vi "Set__slk_mt.vi"(7 "values":string[][](array[string]), 8 "error in (no error)":errorcluster, 11 "digital u32 in":refnum<class "Digital U32__slk_mt.lvclass">) -> (0 "error out":errorcluster, 3 "digital u32 out":refnum<class "Digital U32__slk_mt.lvclass">)   [LabVIEW 2014, in "Lazyboots Menu Tool.lvlib" / "Digital U32__slk_mt.lvclass"]
doc: "Sets the values to the control on GUI.\n\n<b>Values:</b>\n[ [Section, Key, Value], [Section, Key, Value], ..., [Section, Key, Value] ]"
uses:
  Digital U32__slk_mt.lvclass
  Digital U32__slk_mt.lvclass/Digital U32__slk_mt.ctl
panel:
  # "Set__slk_mt.vi\nSets the values to the control on GUI.\n\nNOTICE -- YOU MUST LEAVE THIS NOTICE IN PLACE.\n\nCopyright (c) 2011, LIANG LIU Shawn.Liu.cn@gmail.com\nAll rights reserved.\n\nRedistribution and use in source and binary forms, with or without modification, are permitted provided that the following conditions are met:\n-Redistributions of source code must retain the above copyright notice, this list of conditions and the following disclaimer.\n-Redistributions in binary form must reproduce the above copyright notice, this list of conditions and the following disclaimer in the documentation and/or other materials provided with the distribution.\n-Neither the name of the eLp nor the names of its contributors may be used to endorse or promote products derived from this software without specific prior written permission.\n\nTHIS SOFTWARE IS PROVIDED BY THE COPYRIGHT HOLDERS AND CONTRIBUTORS \"AS IS\" AND ANY EXPRESS OR IMPLIED WARRANTIES, INCLUDING, BUT NOT LIMITED TO, THE IMPLIED WARRANTIES OF MERCHANTABILITY AND FITNESS FOR A PARTICULAR PURPOSE ARE DISCLAIMED. IN NO EVENT SHALL THE COPYRIGHT HOLDER OR CONTRIBUTORS BE LIABLE FOR ANY DIRECT, INDIRECT, INCIDENTAL, SPECIAL, EXEMPLARY, OR CONSEQUENTIAL DAMAGES (INCLUDING, BUT NOT LIMITED TO, PROCUREMENT OF SUBSTITUTE GOODS OR SERVICES; LOSS OF USE, DATA, OR PROFITS; OR BUSINESS INTERRUPTION) HOWEVER CAUSED AND ON ANY THEORY OF LIABILITY, WHETHER IN CONTRACT, STRICT LIABILITY, OR TORT (INCLUDING NEGLIGENCE OR OTHERWISE) ARISING IN ANY WAY OUT OF THE USE OF THIS SOFTWARE, EVEN IF ADVISED OF THE POSSIBILITY OF SUCH DAMAGE."
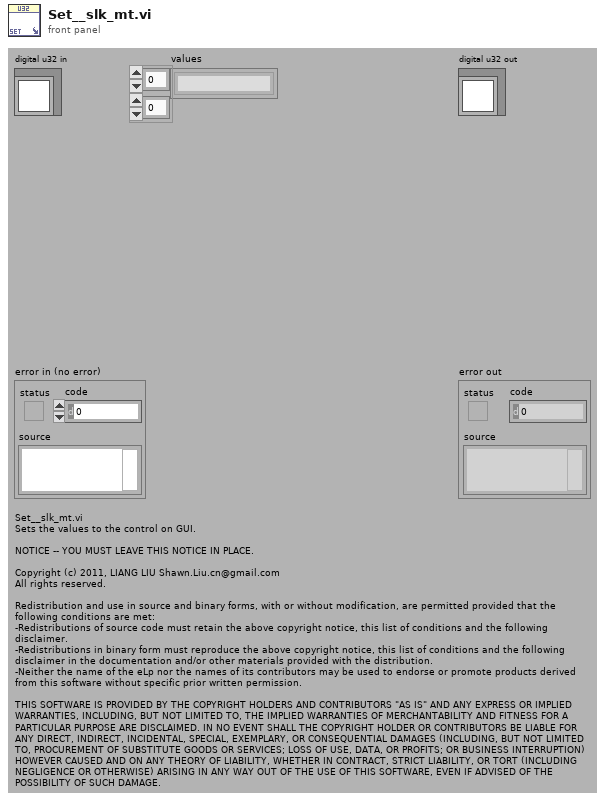
[diagram p1: front panel]
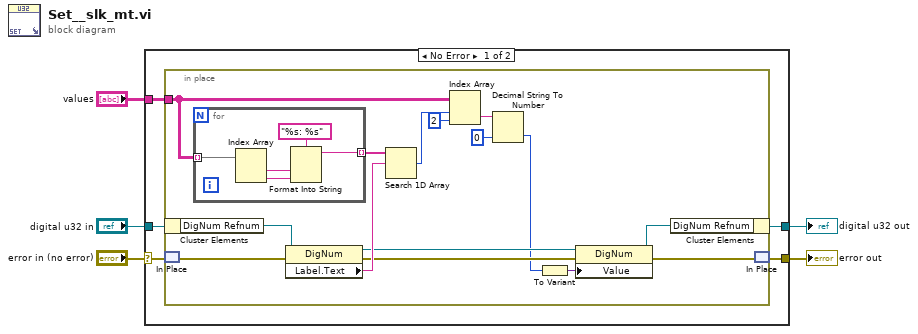
[diagram p0: block diagram]
diagram:
  n1 = case shown="No Error" "error in (no error)" {
    selector: "error in (no error)" -> [w8 w32]
    tunnel: "values" -> [w10 _]
    tunnel: "digital u32 in" -> [w9 w31]
    tunnel: [w7 w32] -> w2
    tunnel: [w6 w31] -> w1
    frame No Error {
      n2 = in-place {
        in-place-border: w10 -> [w15]
        n3 = in-place-cluster #1(w9) -> ("DigNum Refnum"=w14:refnum<vi>)
        n4 = in-place-match #2(w8) -> (w11:errorcluster)
        n5 = for {
          tunnel: w15 -> [w30] mode=indexing
          tunnel: [w26] -> w25 mode=indexing
          n6 = Index Array(array=w30) -> (element #1=w28:string, element #2=w27:string)  [unwired: 2 in]
          n7 = Format Into String(format string="%s: %s", w28, w27) -> (resulting string=w26:string)  [unwired: 2 in, 1 out]
        }
        n8 = property class="DigNum"(reference=w14, error in=w11) -> (reference out=w20:refnum<vi>, error out=w21:errorcluster, "Label.Text"=w24:string)
        n9 = Search 1D Array(1D array=w25, element=w24) -> (index of element=w22:i32)  [unwired: 1 in]
        n10 = Index Array(array=w15, index (row)=w22, index (col)=2 ("disabled index (col)")) -> (element=w19:string)
        n11 = Decimal String To Number(string=w19, default (0L)=u32 0 ("default (0 I32)")) -> (number=w17:u32)  [unwired: 1 in, 1 out]
        n12 = To Variant(anything=w17) -> (Variant=w16:variant)
        n13 = property class="DigNum"(reference=w20, error in=w21, "Value"=w16) -> (reference out=w13:refnum<vi>, error out=w12:errorcluster)
        n14 = in-place-cluster #1("DigNum Refnum"=w13) -> (w6:refnum<class "Digital U32__slk_mt.lvclass">)
        n15 = in-place-match #2(w12) -> (w7:errorcluster)
      }
    }
    frame Error {
    }
  }
  "error out" <- w2
  "digital u32 out" <- w1
